vi "RidgeClassifier.vi"(8 "error in":errorcluster) -> (0 "error out":errorcluster, 3 "out":refnum<class "RidgeClassifier.lvclass">)   [LabVIEW 2020]
doc: "Classifier using Ridge regression.\n\n This classifier first converts the target values into ``{-1, 1}`` and\n then treats the problem as a regression task (multi-output regression in\n the multiclass case).\n\n Read more in the :ref:`User Guide <ridge_regression>`.\n\n Parameters\n ----------\n alpha : float, default=1.0\n Regularization strength; must be a positive float. Regularization\n improves the conditioning of the problem and reduces the variance of\n the estimates. Larger values specify stronger regularization.\n Alpha corresponds to ``1 / (2C)`` in other linear models such as\n :class:`~sklearn.linear_model.LogisticRegression` or\n :class:`~sklearn.svm.LinearSVC`.\n\n fit_intercept : bool, default=True\n Whether to calculate the intercept for this model. If set to false, no\n intercept will be used in calculations (e.g. data is expected to be\n already centered).\n\n normalize : bool, default=False\n This parameter is ignored when ``fit_intercept`` is set to False.\n If True, the regressors X will be normalized before regression by\n subtracting the mean and dividing by the l2-norm.\n If you wish to standardize, please use\n :class:`~sklearn.preprocessing.StandardScaler` before calling ``fit``\n on an estimator with ``normalize=False``.\n\n copy_X : bool, default=True\n If True, X will be copied; else, it may be overwritten.\n\n max_iter : int, default=None\n Maximum number of iterations for conjugate gradient solver.\n The default value is determined by scipy.sparse.linalg.\n\n tol : float, default=1e-3\n Precision of the solution.\n\n class_weight : dict or 'balanced', default=None\n Weights associated with classes in the form ``{class_label: weight}``.\n If not given, all classes are supposed to have weight one.\n\n The \"balanced\" mode uses the values of y to automatically adjust\n weights inversely proportional to class frequencies in the input data\n as ``n_samples / (n_classes * np.bincount(y))``.\n\n solver : {'auto', 'svd', 'cholesky', 'lsqr', 'sparse_cg', 'sag', 'saga'}, default='auto'\n Solver to use in the computational routines:\n\n - 'auto' chooses the solver automatically based on the type of data.\n\n - 'svd' uses a Singular Value Decomposition of X to compute the Ridge\n coefficients. More stable for singular matrices than 'cholesky'.\n\n - 'cholesky' uses the standard scipy.linalg.solve function to\n obtain a closed-form solution.\n\n - 'sparse_cg' uses the conjugate gradient solver as found in\n scipy.sparse.linalg.cg. As an iterative algorithm, this solver is\n more appropriate than 'cholesky' for large-scale data\n (possibility to set `tol` and `max_iter`).\n\n - 'lsqr' uses the dedicated regularized least-squares routine\n scipy.sparse.linalg.lsqr. It is the fastest and uses an iterative\n procedure.\n\n - 'sag' uses a Stochastic Average Gradient descent, and 'saga' uses\n its unbiased and more flexible version named SAGA. Both methods\n use an iterative procedure, and are often faster than other solvers\n when both n_samples and n_features are large. Note that 'sag' and\n 'saga' fast convergence is only guaranteed on features with\n approximately the same scale. You can preprocess the data with a\n scaler from sklearn.preprocessing.\n\n .. versionadded:: 0.17\n Stochastic Average Gradient descent solver.\n .. versionadded:: 0.19\n SAGA solver.\n\n random_state : int, RandomState instance, default=None\n Used when ``solver`` == 'sag' or 'saga' to shuffle the data.\n See :term:`Glossary <random_state>` for details.\n\n Attributes\n ----------\n coef_ : ndarray of shape (1, n_features) or (n_classes, n_features)\n Coefficient of the features in the decision function.\n\n ``coef_`` is of shape (1, n_features) when the given problem is binary.\n\n intercept_ : float or ndarray of shape (n_targets,)\n Independent term in decision function. Set to 0.0 if\n ``fit_intercept = False``.\n\n n_iter_ : None or ndarray of shape (n_targets,)\n Actual number of iterations for each target. Available only for\n sag and lsqr solvers. Other solvers will return None.\n\n classes_ : ndarray of shape (n_classes,)\n The classes labels.\n\n See Also\n --------\n Ridge : Ridge regression.\n RidgeClassifierCV : Ridge classifier with built-in cross validation.\n\n Notes\n -----\n For multi-class classification, n_class classifiers are trained in\n a one-versus-all approach. Concretely, this is implemented by taking\n advantage of the multi-variate response support in Ridge.\n\n \nAvailable methods:\nGet Attributes\nGet Params\nSet Params"
uses:
  RidgeClassifier.lvclass
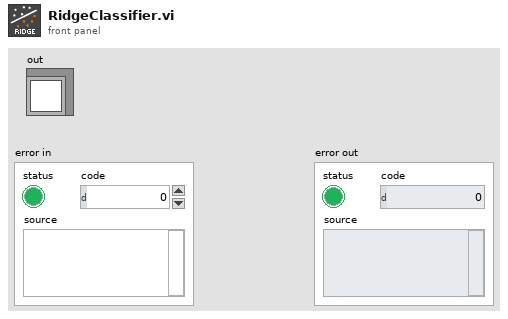
[diagram p1: front panel]
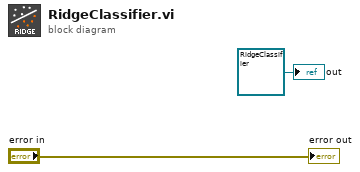
[diagram p0: block diagram]
diagram:
  "out" <- refnum<class "RidgeClassifier.lvclass"> refnum ("model")
  "error out" <- "error in"
